vi "flattenPlaneAngleToXML.vi"   [LabVIEW 2012, in "UnitsAndXML.lvlib"]
doc: "Generates an XML string for <B>planeAngle</B> in the unit specified in <B>planeAngleUnitInXML</B>. Connect <B>planeAngle</B> and <B>planeAngleAgain</B> to the same source. The VI uses <B>planeAngleAgain</B> to obtain the data name."
uses:
  <userlib>/Common/UnitsAndXML/UnitsAndXML.lvlib
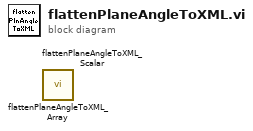
[diagram p0: block diagram]
diagram:
  n1 = call <userlib>:"flattenPlaneAngleToXML_Array.vi"() -> ()  [unwired: 10 in, 2 out]
  n2 = call <userlib>:"flattenPlaneAngleToXML_Scalar.vi"() -> ()  [unwired: 10 in, 2 out]
